vi "Get Axis Properties.vi"(8 "error in":errorcluster, 11 "address":string="192.168.1.101") -> (0 "error out":errorcluster, 2 "Values":string[](array[string]), 3 "Prop Names":string[](array[string]))   [LabVIEW 2017]
panel:
  out "For Documentation Only":string="Content-type: text/plain\n\nroot.ImageSource.I0.Sensor.WhiteBalance=auto\nroot.ImageSource.I0.Sensor.Exposure=auto\nroot.ImageSource.I0.Sensor.ExposurePriority=50\nroot.ImageSource.I0.Sensor.Brightness=60\nroot.ImageSource.I0.Sensor.ColorLevel=50\nroot.ImageSource.I0.Sensor.Sharpness=0\nroot.ImageSource.I0.Sensor.BlacklevelCorrection=0\n"
  out "Camera Request":string
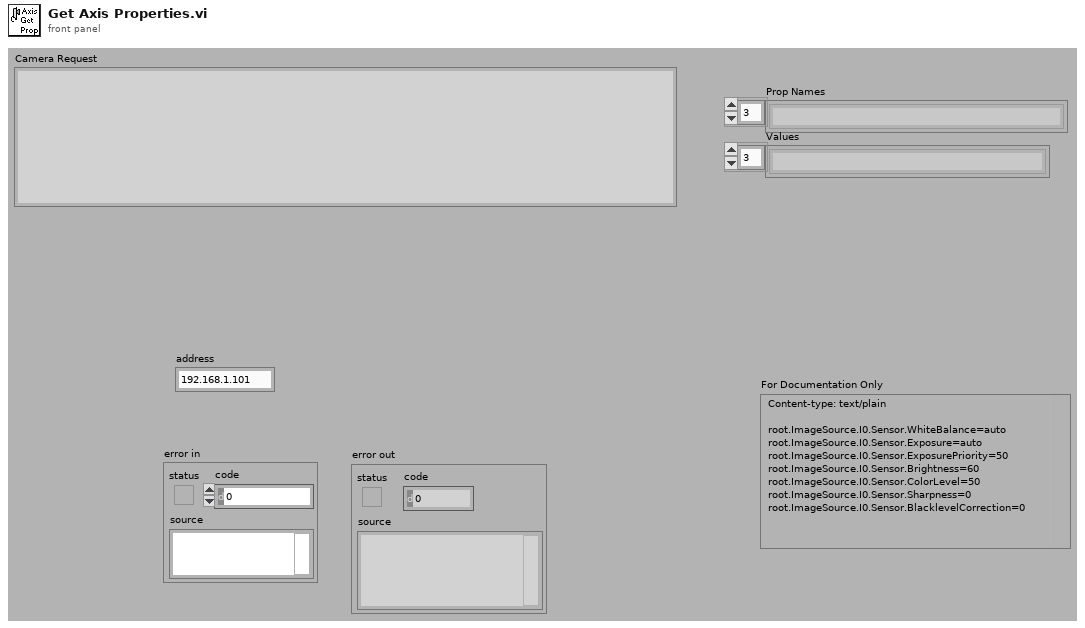
[diagram p1: front panel]
types:
  T1 = enum16{"Standard", "Buffered", "CRLF", "Immediate"}
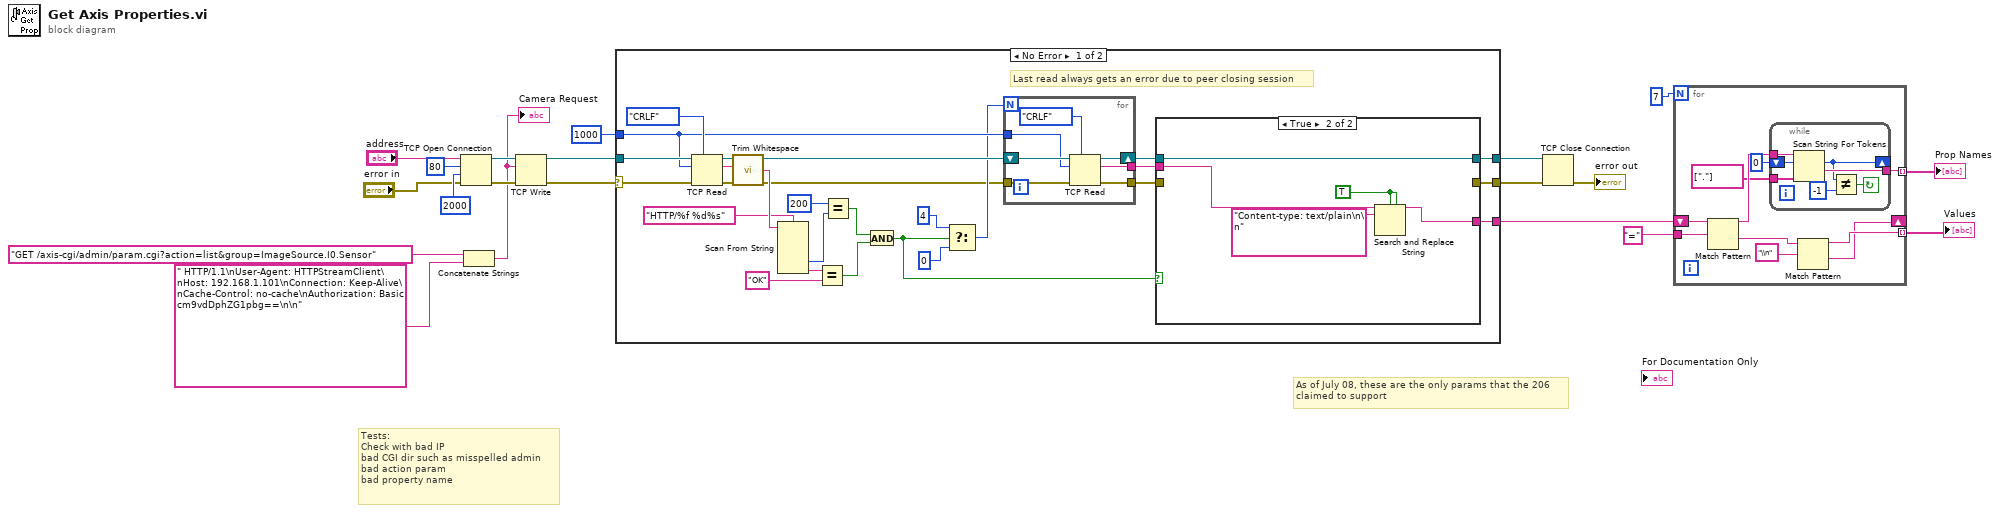
[diagram p0: block diagram]
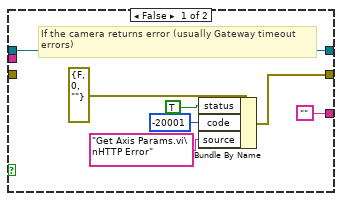
[diagram p2: hidden frame]
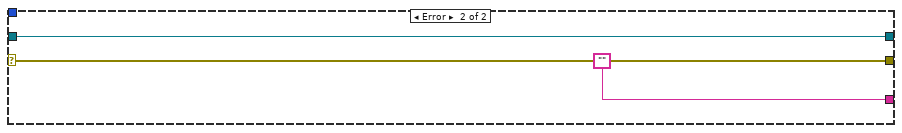
[diagram p3: hidden frame]
diagram:
  # "Tests:\nCheck with bad IP\nbad CGI dir such as misspelled admin\nbad action param\nbad property name"
  # "As of July 08, these are the only params that the 206\nclaimed to support"
  n1 = TCP Open Connection(address="address", remote port or service name=u16 80, timeout ms (60000)=2000, error in (no error)="error in") -> (connection ID=w14:refnum<k5>, error out=w9:errorcluster)  [unwired: 1 in]
  n2 = Concatenate Strings("GET /axis-cgi/admin/param.cgi?action=list&group=ImageSource.I0.Sensor", " HTTP/1.1\nUser-Agent: HTTPStreamClient\nHost: 192.168.1.101\nConnection: Keep-Alive\nCache-Control: no-cache\nAuthorization: Basic cm9vdDphZG1pbg==\n\n") -> (w6:string)
  "Camera Request" <- w6
  n3 = TCP Write(connection ID=w14, data in=w6, error in (no error)=w9) -> (connection ID out=w12:refnum<k5>, error out=w13:errorcluster)  [unwired: 1 in, 1 out]
  n4 = case shown="No Error" w13 {
    selector: w13 -> [w25 w67]
    tunnel: [w45 w67] -> w11
    tunnel: w12 -> [w41 w65]
    tunnel: [w44 ""] -> w5
    tunnel: 1000 ("bytes to read") -> [w30 _]
    tunnel: [w43 w65] -> w7
    frame No Error {
      # "Last read always gets an error due to peer closing session"
      n5 = TCP Read(connection ID=w41, bytes to read=w30, error in (no error)=w25, 7:T1."CRLF" ("mode (standard)")) -> (connection ID out=w31:refnum<k5>, data out=w42:string, error out=w24:errorcluster)  [unwired: 1 in]
      n6 = call <vilib>:"Trim Whitespace.vi"("string"=w42) -> ("trimmed string"=w39:string)  [unwired: 1 in]
      n7 = Scan From String(format string="HTTP/%f %d%s", input string=w39) -> (output 2=w37:i32, output 3=w35:string)  [unwired: 6 in, 3 out]
      n8 = Equal?(x=w35, y="OK" ("format string")) -> (x = y?=w33:bool)
      n9 = Equal?(x=200, y=w37) -> (x = y?=w32:bool)
      n10 = And(x=w32, y=w33) -> (x .and. y?=w22:bool)
      n11 = Select(t=4, s=w22, f=0) -> (s? t:f=w27:i32)
      n12 = for {
        N: w27 -> [_]
        tunnel: w30 -> [w50]
        tunnel: [w49] -> w21
        shift-right: [w48] -> w26
        shift-left: w31 -> [w51]
        tunnel: w24 -> [w47]
        tunnel: [w46] -> w23
        n13 = TCP Read(connection ID=w51, bytes to read=w50, error in (no error)=w47, 7:T1."CRLF" ("mode (standard)")) -> (connection ID out=w48:refnum<k5>, data out=w49:string, error out=w46:errorcluster)  [unwired: 1 in]
      }
      n14 = case shown="True" w22 {
        tunnel: w26 -> [w53 w64]
        tunnel: w23 -> [_ _]
        tunnel: [w59 _] -> w45
        tunnel: ["" w61] -> w44
        tunnel: [w53 w64] -> w43
        tunnel: w21 -> [_ w62]
        frame False {
          # "If the camera returns error (usually Gateway timeout\nerrors)"
          n15 = Bundle By Name(cluster=errorcluster {"status"=FALSE, "code"=0, "source"=""} ("error in"), "status"=TRUE, "code"=-20001, "source"="Get Axis Params.vi\nHTTP Error") -> (w59:errorcluster)
        }
        frame True {
          w60 = TRUE ("ignore case? (F)")
          n16 = Search and Replace String(case sensitive?=w60, multiline?=w60, input string=w62, search string="Content-type: text/plain\n\n" ("regular expression")) -> (result string=w61:string)  [unwired: 4 in, 3 out]
        }
      }
    }
    frame Error {
    }
  }
  n17 = TCP Close Connection(connection ID=w7, error in (no error)=w11) -> (error out=→"error out":errorcluster)  [unwired: 1 in, 1 out]
  n18 = for {
    N: 7 -> [_]
    tunnel: "=" ("regular expression") -> [w76]
    tunnel: [w74] -> w3 mode=indexing
    shift-right: [w72] -> _
    shift-left: w5 -> [w77]
    tunnel: [w69] -> w1 mode=indexing
    n19 = Match Pattern(string=w77, regular expression=w76) -> (before substring=w71:string, after substring=w73:string)  [unwired: 1 in, 2 out]
    n20 = while {
      tunnel: w71 -> [w84]
      tunnel: string[] ["."] ("delimiters (\\s,\\t,\\r,\\n)") -> [w83]
      tunnel: [w80] -> w69
      shift-right: [w78] -> _
      shift-left: 0 ("offset past token") -> [w79]
      stop <- w81 continue-if-true
      n21 = Scan String For Tokens(6:w83, 8:w79, 9:w84) -> (1:w80:string, 2:w78:i32)  [unwired: 3 in, 2 out]
      n22 = Not Equal?(x=w78, y=-1) -> (x != y?=w81:bool)
    }
    n23 = Match Pattern(string=w73, regular expression="\\n") -> (before substring=w74:string, after substring=w72:string)  [unwired: 1 in, 2 out]
  }
  "Prop Names" <- w1
  "Values" <- w3
